vi "未命名 1.vi"() -> ()   [LabVIEW 2019]
panel:
  out "数值 2":dbl
  in  "数值":dbl
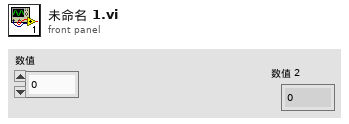
[diagram p1: front panel]
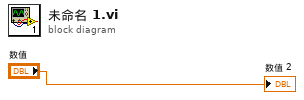
[diagram p0: block diagram]
diagram:
  "数值 2" <- "数值"
